vi "start.vi"(8 "error in (no error)":errorcluster, 11 "WinX32Camera in":refnum<class "WinX32Camera.lvclass">) -> (0 "error out":errorcluster, 3 "WinX32Camera out":refnum<class "WinX32Camera.lvclass">)   [LabVIEW 2011, in "WinX32Camera.lvclass"]
uses:
  WinX32Camera.lvclass
  WinX32Camera.lvclass/WinX32Camera.ctl
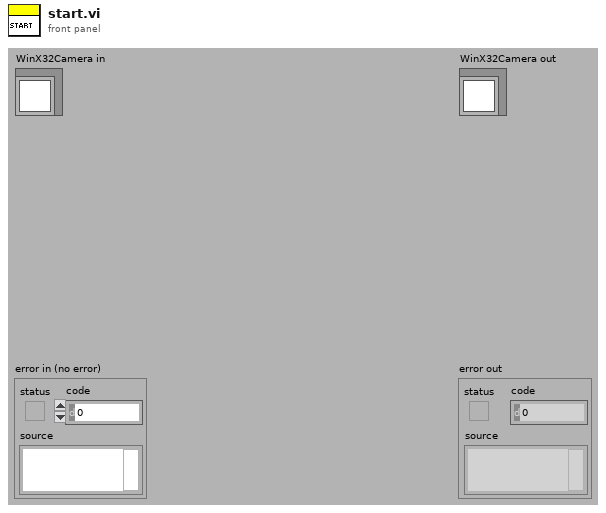
[diagram p1: front panel]
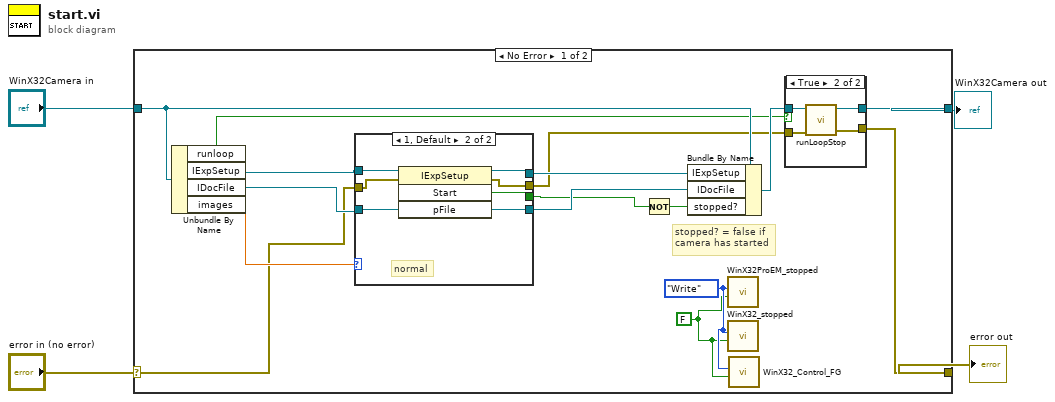
[diagram p0: block diagram]
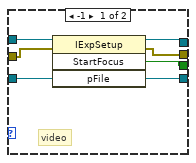
[diagram p3: hidden frame]
diagram:
  n1 = case shown="No Error" "error in (no error)" {
    selector: "error in (no error)" -> [w12 w42]
    tunnel: [w9 w42] -> w3
    tunnel: [w8 w41] -> w1
    tunnel: "WinX32Camera in" -> [w20 w41]
    frame No Error {
      w5 = FALSE
      w6 = enum16{"Write", "Read"}."Write" ("Action")
      # "stopped? = false if\ncamera has started"
      n2 = Unbundle By Name(w20) -> ("runloop"=w7:bool, "IExpSetup"=w14:refnum<k7>, "IDocFile"=w13:refnum<k7>, "images"=w18:dbl)
      n3 = case shown="1, Default" w18 {
        tunnel: w14 -> [w33 w40]
        tunnel: w13 -> [w28 w35]
        tunnel: [w31 w38] -> w17
        tunnel: w12 -> [w29 w36]
        tunnel: [w30 w37] -> w10
        tunnel: [w32 w39] -> w19
        tunnel: [w27 w34] -> w15
        frame -1 {
          # "video"
          n4 = invoke class="IExpSetup" method="StartFocus"(reference=w33, error in=w29, "pFile"=w28) -> (reference out=w32:refnum<k7>, error out=w30:errorcluster, "StartFocus"=w27:bool, "pFile"=w31:refnum<k7>)  [unwired: 1 in]
        }
        frame 1, Default {
          # "normal"
          n5 = invoke class="IExpSetup" method="Start"(reference=w40, error in=w36, "pFile"=w35) -> (reference out=w39:refnum<k7>, error out=w37:errorcluster, "Start"=w34:bool, "pFile"=w38:refnum<k7>)  [unwired: 1 in]
        }
      }
      n6 = Not(x=w15) -> (.not. x?=w16:bool)
      n7 = Bundle By Name(cluster=w20, "IExpSetup"=w19, "IDocFile"=w17, "stopped?"=w16) -> (w11:refnum<class "WinX32Camera.lvclass">)
      n8 = call "WinX32ProEM_stopped.vi"("stop"=w5, "Action"=w6) -> ()  [unwired: 9 in, 1 out]
      n9 = call "WinX32_stopped.vi"("stop"=w5, "Action"=w6) -> ()  [unwired: 9 in, 1 out]
      n10 = call "WinX32_Control_FG.vi"("stop"=w5, "Action"=w6) -> ()  [unwired: 9 in, 1 out]
      n11 = case shown="True" w7 {
        tunnel: w11 -> [w22 w26]
        tunnel: w10 -> [w21 w25]
        tunnel: [w21 w24] -> w9
        tunnel: [w22 w23] -> w8
        frame False {
        }
        frame True {
          n12 = call "runLoopStop.vi"("error in (no error)"=w25, "WinX32Camera in"=w26) -> ("error out"=w24:errorcluster, "WinX32Camera out"=w23:refnum<class "WinX32Camera.lvclass">)  [unwired: 8 in]
        }
      }
    }
    frame Error {
    }
  }
  "error out" <- w3
  "WinX32Camera out" <- w1
